vi "add_lookup_event_listener.vi"(6 "id (unnamed)":string, 8 "error in (no error)":errorcluster, 9 "user event":refnum<user-event>, 10 "Base Class (LabVIEW Object)":refnum<class>, 11 "Mapped Lookup in":refnum<class "Mapped Lookup.lvclass">) -> (0 "error out":errorcluster, 3 "Mapped Lookup out":refnum<class "Mapped Lookup.lvclass">)   [LabVIEW 2019, in "LVCOOOP.lvlib" / "Lookup API.lvlib" / "Mapped Lookup.lvclass"]
uses:
  Mapped Lookup.lvclass
  Mapped Lookup.lvclass/Mapped Lookup.ctl
  <vilib>/Utility/miscctls.llb/LVMapReplaceAction.ctl
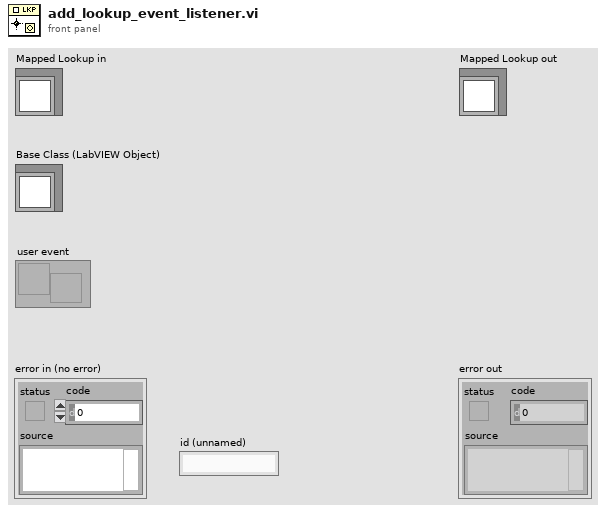
[diagram p1: front panel]
types:
  T1 = typedef "LVMapReplaceAction.ctl" = enum32{"Modify Entry only if found", "Add or Modify Entry", "Delete Entry"}
  T2 = map{string, cluster{"instances":refnum<data-value>, "events":refnum<data-value>}}
  T3 = cluster{"instances":refnum<data-value>, "events":refnum<data-value>}
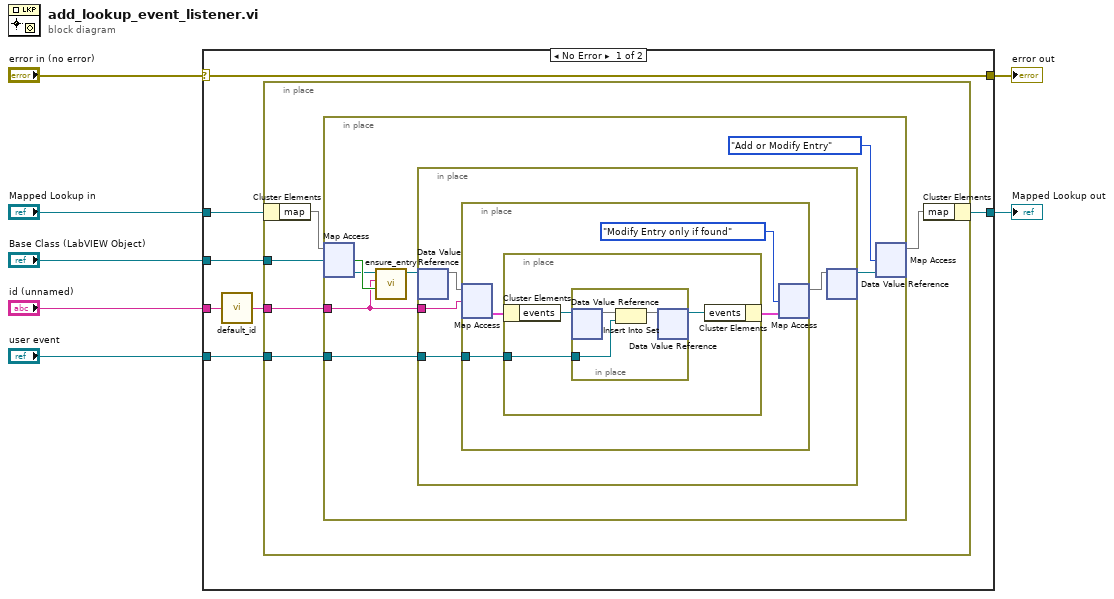
[diagram p0: block diagram]
diagram:
  n1 = case shown="No Error" "error in (no error)" {
    selector: "error in (no error)" -> [w14 w42]
    tunnel: [w14 w42] -> w1
    tunnel: [w8 w41] -> w2
    tunnel: "Mapped Lookup in" -> [w13 w41]
    tunnel: "Base Class (LabVIEW Object)" -> [w12 _]
    tunnel: "id (unnamed)" -> [w11 _]
    tunnel: "user event" -> [w9 _]
    frame No Error {
      n2 = call "default_id.vi"("id (unnamed)"=w11) -> ("String"=w10:string)
      n3 = in-place {
        in-place-border: w12 -> [w15]
        in-place-border: w10 -> [w19]
        in-place-border: w9 -> [w18]
        n4 = in-place-cluster #1(w13) -> ("map"=w17:map{refnum<class>, refnum<data-value>})
        n5 = in-place {
          in-place-border: w19 -> [w21]
          in-place-border: w18 -> [w24]
          n6 = in-place-map #2(w17, w15) -> (w23:refnum<data-value>, w25:bool)  [unwired: 1 in]
          n7 = call "ensure_entry.vi"("not found?"=w25, "id"=w21, "named entries in"=w23) -> ("named entries out"=w22:refnum<data-value>)  [unwired: 8 in]
          n8 = in-place {
            in-place-border: w24 -> [w30]
            in-place-border: w21 -> [w28]
            n9 = in-place-dvr #3(w22) -> (w29:T2)  [unwired: 1 out]
            n10 = in-place {
              in-place-border: w30 -> [w34]
              n11 = in-place-map #4(w29, w28) -> (w33:T3)  [unwired: 1 in, 1 out]
              n12 = in-place {
                in-place-border: w34 -> [w37]
                n13 = in-place-cluster #5(w33) -> ("events"=w36:refnum<data-value>)
                n14 = in-place {
                  in-place-border: w37 -> [w39]
                  n15 = in-place-dvr #6(w36) -> (w40:set{refnum<user-event>})  [unwired: 1 out]
                  n16 = Insert Into Set(10:w39, 11:w40) -> (3:w38:set{refnum<user-event>})  [unwired: 1 out]
                  n17 = in-place-dvr #6(w38) -> (w35:refnum<data-value>)  [unwired: 1 out]
                }
                n18 = in-place-cluster #5("events"=w35) -> (w32:T3)
              }
              n19 = in-place-map #4(w32, LVMapReplaceAction."Modify Entry only if found" ("action")) -> (w27:T2)  [unwired: 2 out]
            }
            n20 = in-place-dvr #3(w27) -> (w20:refnum<data-value>)  [unwired: 1 out]
          }
          n21 = in-place-map #2(w20, LVMapReplaceAction."Add or Modify Entry" ("action")) -> (w16:map{refnum<class>, refnum<data-value>})  [unwired: 2 out]
        }
        n22 = in-place-cluster #1("map"=w16) -> (w8:refnum<class "Mapped Lookup.lvclass">)
      }
    }
    frame Error {
    }
  }
  "error out" <- w1
  "Mapped Lookup out" <- w2
